vi "autobox.vi"() -> (0 "autobox switches":cluster{bool, bool, bool})   [LabVIEW 2011]
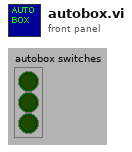
[diagram p1: front panel]
types:
  T1 = typedef "WPI_AnalogChannelDevRef.ctl" = cluster{"DevStatus":errorcluster, "Analog Module":T2, "Analog Channel":T3}
  T2 = typedef "FPGA_TypedefAnalogModule.ctl" = enum16{"Analog Module 1", "Analog Module 2"}
  T3 = typedef "FPGA_AIChannel.ctl" = enum8{"AI 1", "AI 2", "AI 3", "AI 4", "AI 5", "AI 6", "AI 7", "AI 8", "Invalid"}
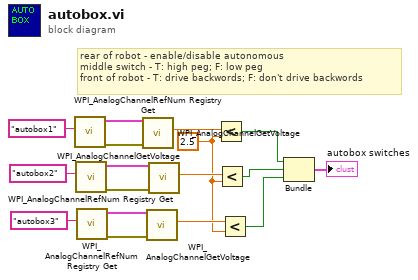
[diagram p0: block diagram]
diagram:
  w2 = 2.5 ("y")
  # "rear of robot - enable/disable autonomous\nmiddle switch - T: high peg; F: low peg\nfront of robot - T: drive backwords; F: don't drive backwords"
  n1 = call <vilib>:"WPI_AnalogChannelRefNum Registry Get.vi"("refnum name"="autobox1") -> ("error out"=w13:errorcluster, "AIDeviceRef"=w14:T1)  [unwired: 1 in, 8 out]
  n2 = call <vilib>:"WPI_AnalogChannelRefNum Registry Get.vi"("refnum name"="autobox2") -> ("error out"=w11:errorcluster, "AIDeviceRef"=w12:T1)  [unwired: 1 in, 8 out]
  n3 = call <vilib>:"WPI_AnalogChannelRefNum Registry Get.vi"("refnum name"="autobox3") -> ("error out"=w9:errorcluster, "AIDeviceRef"=w10:T1)  [unwired: 1 in, 8 out]
  n4 = call <vilib>:"WPI_AnalogChannelGetVoltage.vi"("error in (no error)"=w13, "AIDeviceRef"=w14) -> ("Voltage"=w5:dbl)  [unwired: 9 out]
  n5 = call <vilib>:"WPI_AnalogChannelGetVoltage.vi"("error in (no error)"=w9, "AIDeviceRef"=w10) -> ("Voltage"=w3:dbl)  [unwired: 9 out]
  n6 = call <vilib>:"WPI_AnalogChannelGetVoltage.vi"("error in (no error)"=w11, "AIDeviceRef"=w12) -> ("Voltage"=w4:dbl)  [unwired: 9 out]
  n7 = Less?(x=w5, y=w2) -> (x < y?=w6:bool)
  n8 = Less?(x=w4, y=w2) -> (x < y?=w7:bool)
  n9 = Less?(x=w3, y=w2) -> (x < y?=w8:bool)
  n10 = Bundle(w6, w7, w8) -> (→"autobox switches":cluster{bool, bool, bool})  [unwired: 1 out]
